vi "通知器的用法.vi"() -> ()   [LabVIEW 2010]
panel:
  out "数值":dbl
  in  "停止":bool
  in  "暂停循环":bool
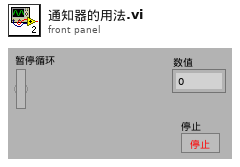
[diagram p1: front panel]
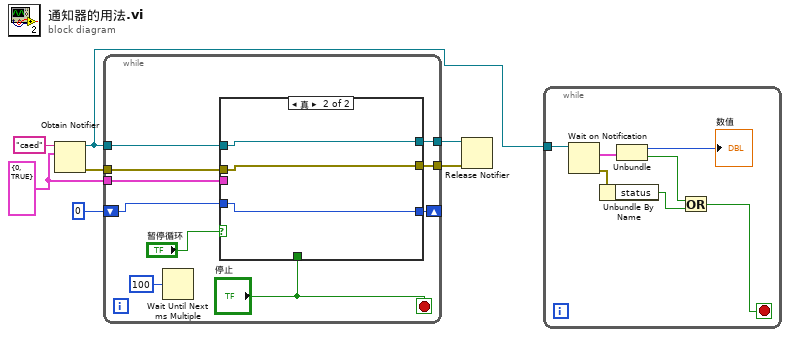
[diagram p0: block diagram]
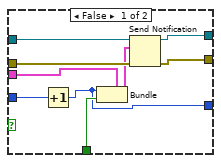
[diagram p2: hidden frame]
diagram:
  w5 = cluster{i32, bool} {0, TRUE}
  n1 = Obtain Notifier(name (unnamed)="caed" ("名称（未命名）"), notification data type=w5) -> (notifier out=w2:refnum<notifier>, error out=w6:errorcluster)  [unwired: 2 in, 1 out]
  n2 = while {
    tunnel: w2 -> [w16]
    tunnel: w6 -> [w15]
    tunnel: w5 -> [w13]
    tunnel: [w12] -> w4
    tunnel: [w11] -> w3
    shift-right: [w8] -> _
    shift-left: 0 -> [w9]
    stop <- "停止" stop-if-true
    n3 = Wait Until Next ms Multiple(millisecond multiple=u32 100 ("毫秒倍数")) -> ()  [unwired: 1 out]
    n4 = case shown="真" "暂停循环" {
      tunnel: w16 -> [w26 w29]
      tunnel: w15 -> [w25 w28]
      tunnel: "停止" -> [w24 _]
      tunnel: w13 -> [w22 _]
      tunnel: [w21 w29] -> w12
      tunnel: [w20 w28] -> w11
      tunnel: w9 -> [w19 w27]
      tunnel: [w18 w27] -> w8
      frame False {
        n5 = Increment(x=w19) -> (x+1=w18:i32)
        n6 = Bundle(cluster=w22, w18, w24) -> (w23:cluster{i32, bool})
        n7 = Send Notification(notification=w23, notifier=w26, error in (no error)=w25) -> (notifier out=w21:refnum<notifier>, error out=w20:errorcluster)
      }
      frame True {
      }
    }
  }
  n8 = Release Notifier(notifier=w4, error in (no error)=w3) -> ()  [unwired: 1 in, 3 out]
  n9 = while {
    tunnel: w2 -> [w36]
    stop <- w31 stop-if-true
    n10 = Wait on Notification(notifier=w36) -> (notification=w35:cluster{i32, bool}, error out=w34:errorcluster)  [unwired: 3 in, 2 out]
    n11 = Unbundle By Name(w34) -> ("status"=w32:bool)
    n12 = Unbundle(w35) -> (→"数值":i32, w33:bool)
    n13 = Or(x=w33, y=w32) -> (x .or. y?=w31:bool)
  }
